vi "new itc and dmm file.vi"() -> ()   [LabVIEW 2009]
panel:
  out "Waveform Chart":dynamicdata(graph)
  out "Sensors Resistance":dynamicdata(graph)
  out "All Temp Sensor":dynamicdata(graph) caption="All temp Chart"
  out "Measurement":bool caption="Taken"
  in  "stop":bool
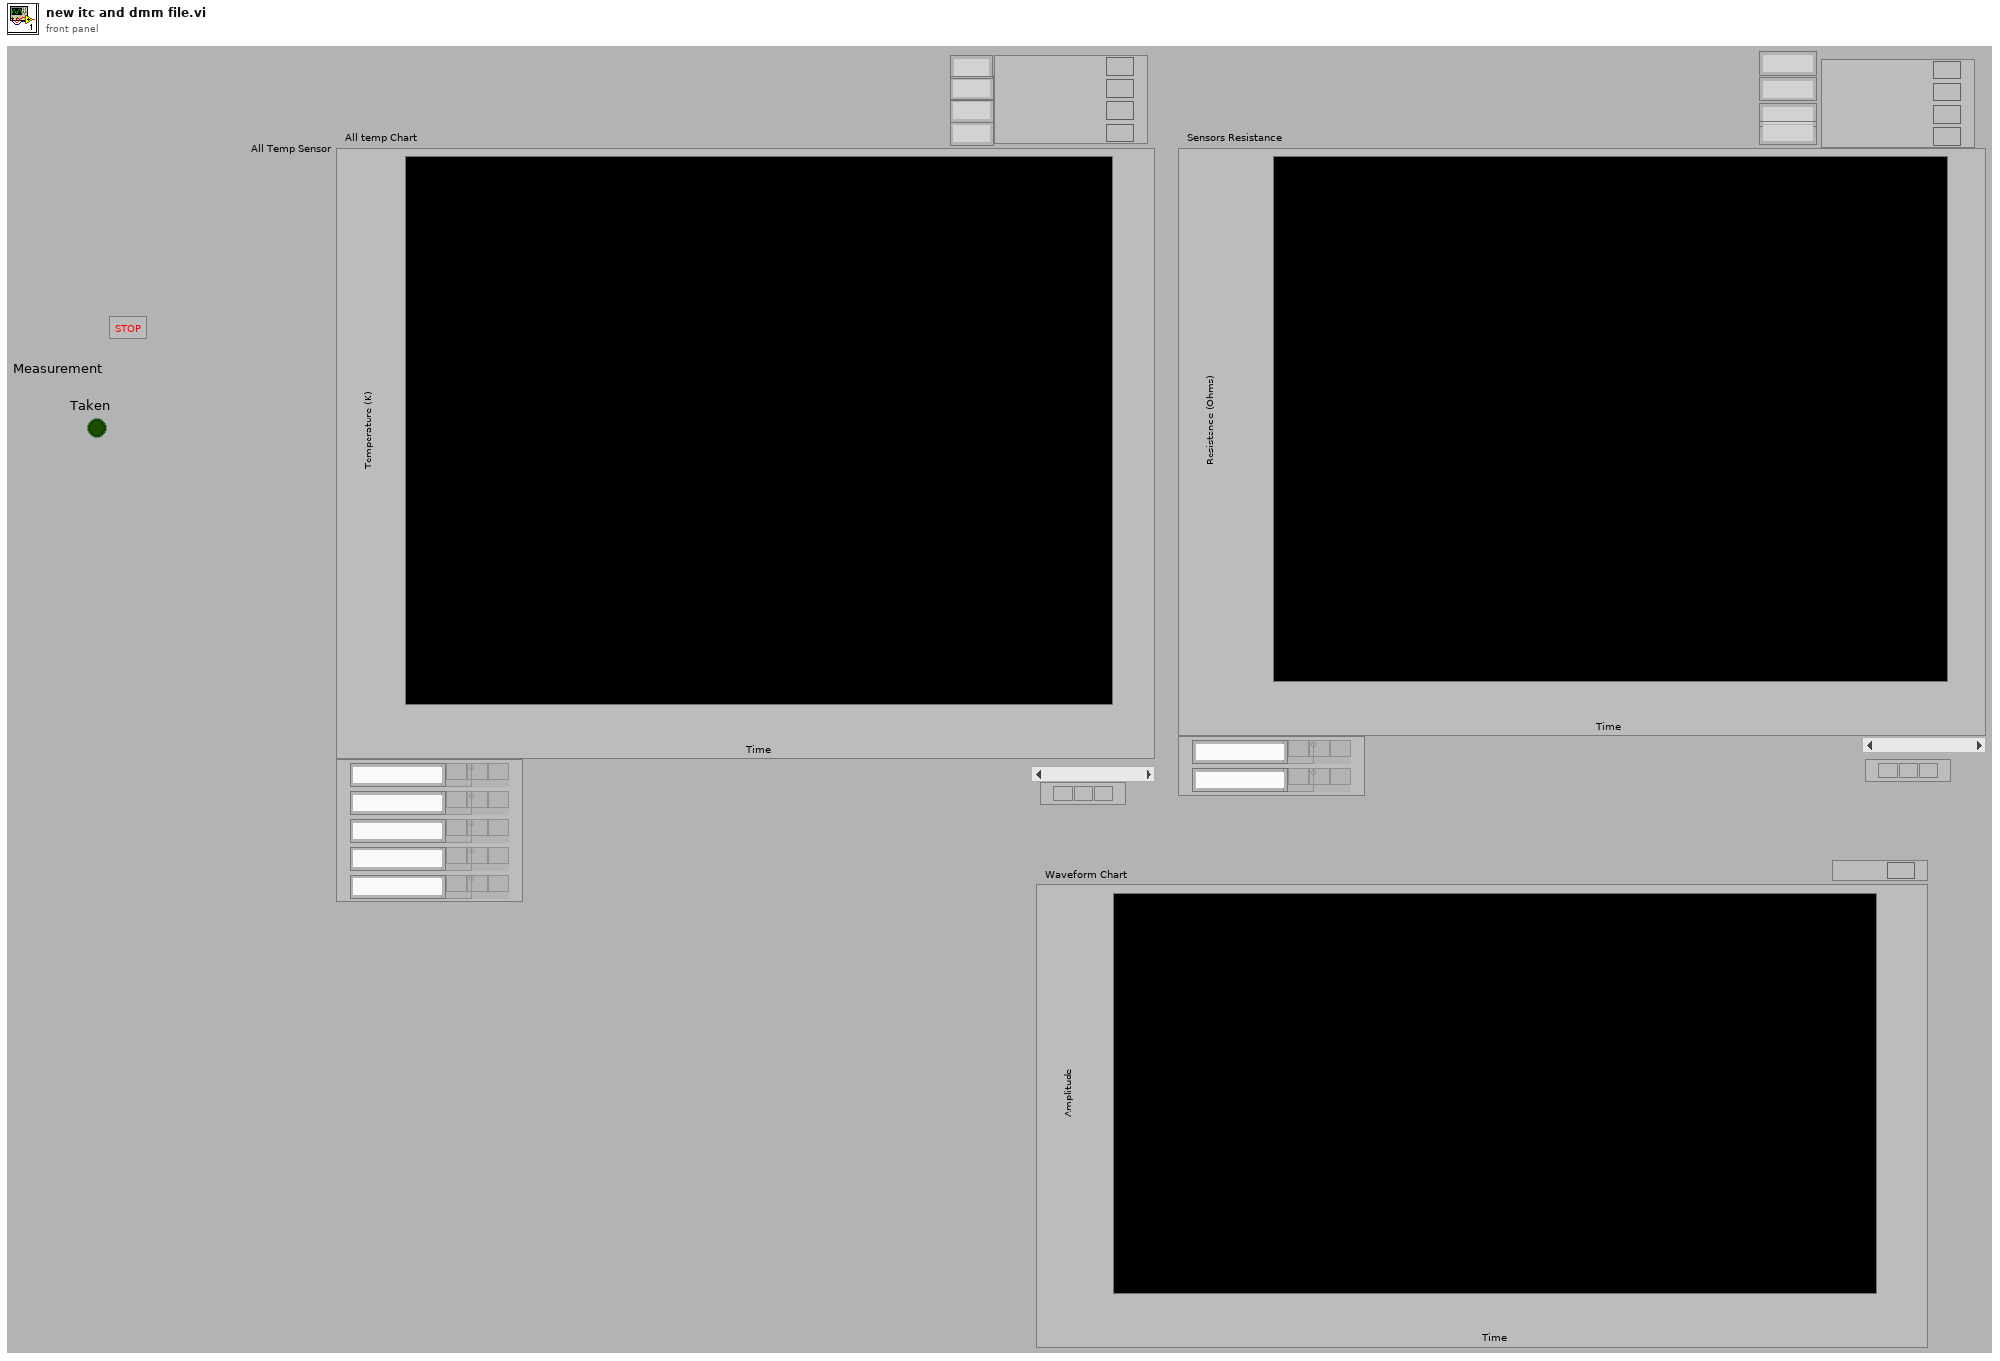
[diagram p1: front panel]
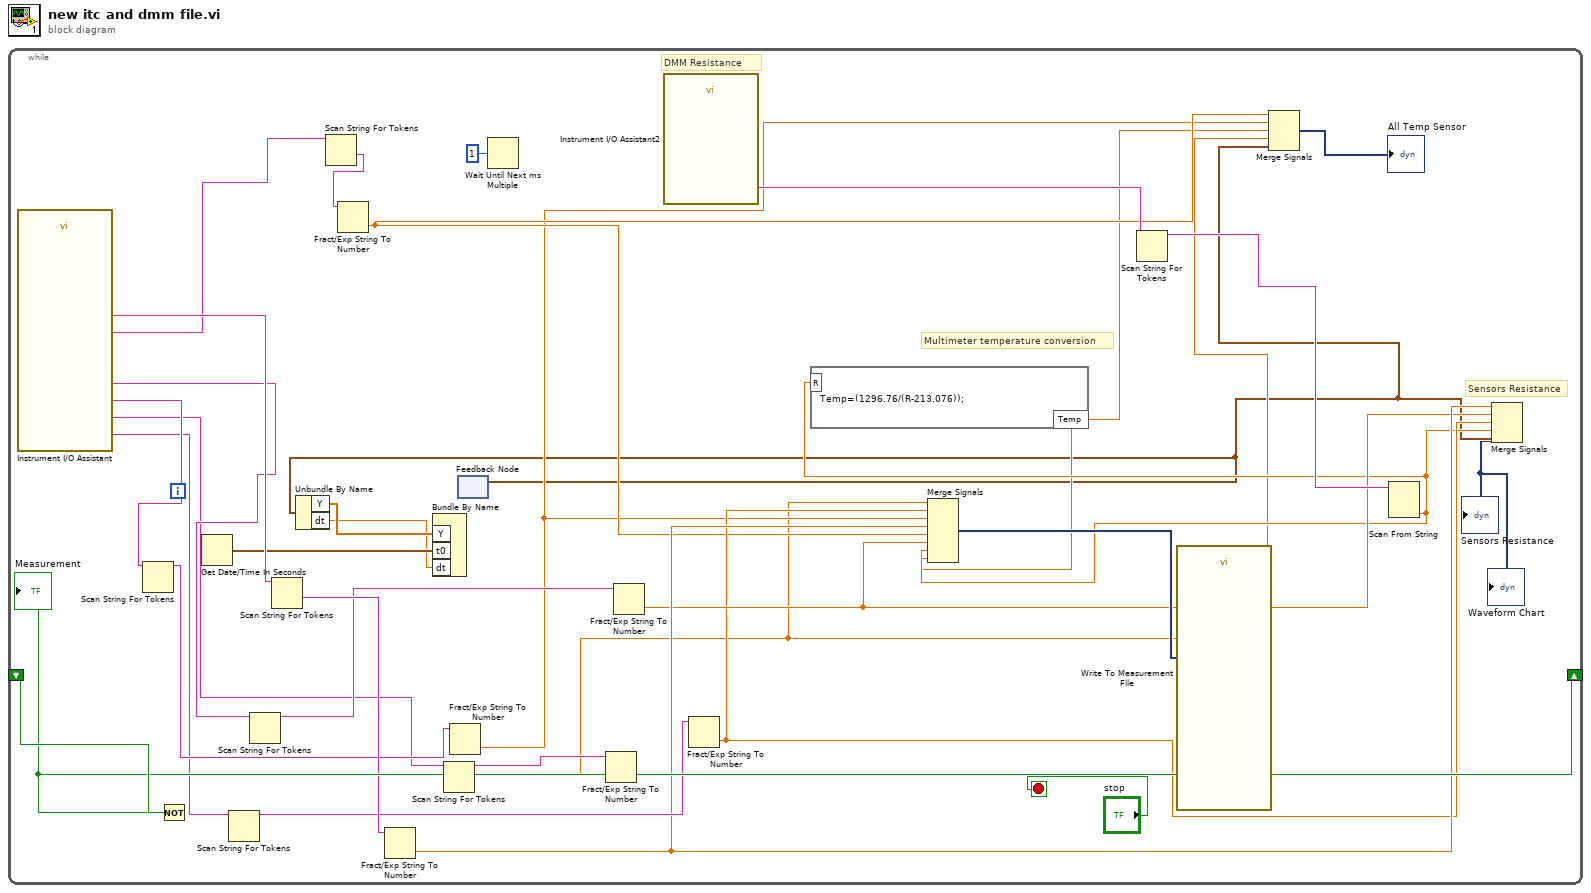
[diagram p0: block diagram]
diagram:
  n1 = while {
    shift-right: [w33] -> _
    shift-left: _ -> [w34]
    stop <- "stop" stop-if-true
    # "DMM Resistance"
    # "Sensors Resistance"
    # "Multimeter temperature conversion"
    n2 = call "Instrument I/O Assistant"() -> ("CCS Resistance"=w22:string, "CCS Temperature"=w20:string, "Allen Bradley Temperature"=w24:string, "Allen Bradley Resistance"=w26:string, "Cernox Temp"=w30:string, "Cernox Resistance"=w32:string)  [unwired: 21 in, 1 out]
    n3 = Scan String For Tokens(9:w24) -> (3:w23:string)  [unwired: 5 in, 3 out]
    n4 = Not(x=w34) -> (.not. x?=w33:bool)
    "Measurement" <- w33
    n5 = Get Date/Time In Seconds() -> (seconds since 1Jan1904=w27:timestamp)
    n6 = Scan String For Tokens(9:w22) -> (3:w21:string)  [unwired: 5 in, 3 out]
    n7 = Scan String For Tokens(9:w26) -> (3:w25:string)  [unwired: 5 in, 3 out]
    n8 = Scan String For Tokens(9:w32) -> (1:w31:string)  [unwired: 5 in, 3 out]
    n9 = Scan String For Tokens(9:w30) -> (1:w28:string)  [unwired: 5 in, 3 out]
    n10 = Fract/Exp String To Number(string=w28) -> (number=w10:dbl)  [unwired: 3 in, 1 out]
    n11 = Fract/Exp String To Number(string=w31) -> (number=w14:dbl)  [unwired: 3 in, 1 out]
    n12 = Scan String For Tokens(9:w20) -> (3:w19:string)  [unwired: 5 in, 3 out]
    n13 = Fract/Exp String To Number(string=w23) -> (number=w9:dbl)  [unwired: 3 in, 1 out]
    n14 = feedback #1() -> (w2:waveform(dbl))  [unwired: 1 in]
    n15 = Unbundle By Name(w2) -> ("Y"=w5:dbl[], "dt"=w4:dbl)
    n16 = Bundle By Name("Y"=w5, "t0"=w27, "dt"=w4) -> (w3:waveform(dbl))  [unwired: 1 in]
    n17 = Wait Until Next ms Multiple(millisecond multiple=u32 1) -> ()  [unwired: 1 out]
    n18 = Fract/Exp String To Number(string=w19) -> (number=w8:dbl)  [unwired: 3 in, 1 out]
    n19 = Fract/Exp String To Number(string=w25) -> (number=w13:dbl)  [unwired: 3 in, 1 out]
    n20 = call "Instrument I/O Assistant2"() -> ("Sample rate"=w15:string)  [unwired: 26 in, 1 out]
    n21 = Fract/Exp String To Number(string=w21) -> (number=w12:dbl)  [unwired: 3 in, 1 out]
    n22 = Scan String For Tokens(9:w15) -> (3:w16:string)  [unwired: 5 in, 3 out]
    n23 = Scan From String(input string=w16) -> (output 1=w11:dbl)  [unwired: 4 in, 3 out]
    n24 = formula code="Temp=(1296.76/(R-213.076));"("R"=w11) -> ("Temp"=w7:dbl)
    n25 = Merge Signals(w8, w12, w9, w14, w10, w13, w11, w7) -> (w29:dynamicdata)
    n26 = call "Write To Measurement File"("Signals"=w29) -> ()  [unwired: 16 in, 3 out]
    n27 = Merge Signals(w10, w9, w7, w8, w2) -> (→"All Temp Sensor":dynamicdata)
    n28 = Merge Signals(w14, w13, w12, w11, w2) -> (→"Sensors Resistance" →"Waveform Chart":dynamicdata)
  }
